vi "CIC FXPi18x1.vi"(0 "input":fxp<+/-,18,1>, 1 "reset":bool, 5 "decimation factor":fxp<+,16,16>, 7 "config valid":bool, 9 "input valid":bool) -> (4 "output":fxp<+/-,64,1>, 10 "output valid":bool)   [LabVIEW 2018, in "Lock-In Amplifier Example FPGA.lvlib"]
uses:
  Lock-In Amplifier Example FPGA.lvlib
  <vilib>/rvi/XilinxIP/XIPIN_XNode/niFpgaXIPIN.xnode
  Private/cic/xsim.dir/cic_0EFBEBF2FBC14C9D8ACC94B2504D3B1A/xsimk_0EFBEBF2FBC14C9D8ACC94B2504D3B1A.dll
  <vilib>/rvi/IPIntegrationNode/IPINode_Xnode/niFpgaIPINode.xnode
  <vilib>/rvi/IPIntegrationNode/IPINode_Typedef/niFpgaIPINodeSupportedFamilies.ctl
  <vilib>/rvi/IPIntegrationNode/IPINode_Utilities/niFpgaIPINodeSimCore.vi
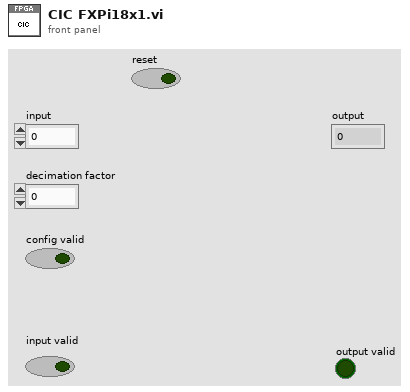
[diagram p1: front panel]
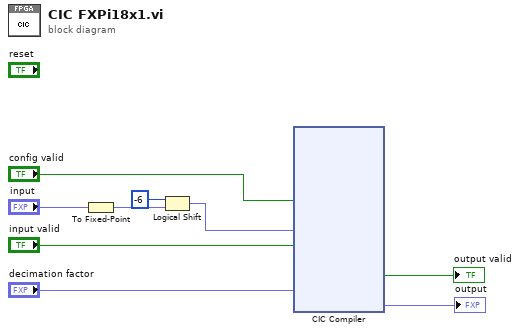
[diagram p0: block diagram]
diagram:
  n1 = To Fixed-Point(number="input") -> (fixed-point=w3:fxp<+/-,24,1>)  [unwired: 1 in]
  n2 = Logical Shift(y=i16 -6, x=w3) -> (x << y=w2:fxp<+/-,24,1>)
  n3 = xnode ("CIC Compiler")("s_axis_config_tvalid"="config valid", "s_axis_data_tdata"=w2, "s_axis_data_tvalid"="input valid", "s_axis_config_tdata"="decimation factor") -> ("m_axis_data_tvalid"=→"output valid":bool, "m_axis_data_tdata"=→"output":fxp<+/-,64,1>)  [unwired: 2 out]
